vi "TDMS Channel Name.vi"(8 "error in":errorcluster, 11 "channel number":u16) -> (0 "error out":errorcluster, 3 "channel name":string)   [LabVIEW 2011]
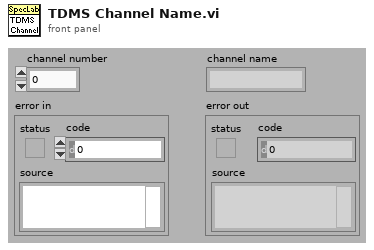
[diagram p1: front panel]
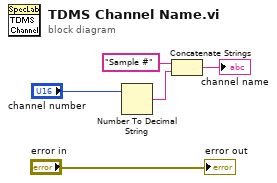
[diagram p0: block diagram]
diagram:
  n1 = Number To Decimal String(number="channel number") -> (decimal integer string=w5:string)  [unwired: 1 in]
  n2 = Concatenate Strings("Sample #" ("string"), w5) -> (→"channel name":string)
  "error out" <- "error in"
